vi "Configuration Window.vi"(8 "error in (no error)":errorcluster, 11 "DB Ref":refnum<class "SharedData.lvclass">) -> (0 "error out":errorcluster, 3 "DB Ref (dup)":refnum<class "SharedData.lvclass">)   [LabVIEW 2014]
uses:
  <vilib>/NEVSTOP/Shared Data Library/SharedData/SharedData.lvclass
  <vilib>/NEVSTOP/Shared Data Library/SharedData/SharedData.lvclass/SharedData.ctl
  <vilib>/NEVSTOP/Shared Data Library/SharedData/Data operation/_int32.vi
  <vilib>/NEVSTOP/Shared Data Library/SharedData/Data operation/_variant.vi
  <vilib>/NEVSTOP/Shared Data Library/SharedData/support/_[error50002]Invalid DataType.vi
  <vilib>/NEVSTOP/Shared Data Library/SharedData/support/_[error50001]Can't Found Value.vi
  <vilib>/NEVSTOP/Shared Data Library/SharedData/support/_[error50000]Invalid DB REF.vi
  <vilib>/Utility/error.llb/Trim Whitespace.vi
panel:
  in  "Display Time(ms)":i32 min=0 max=10000 step=100
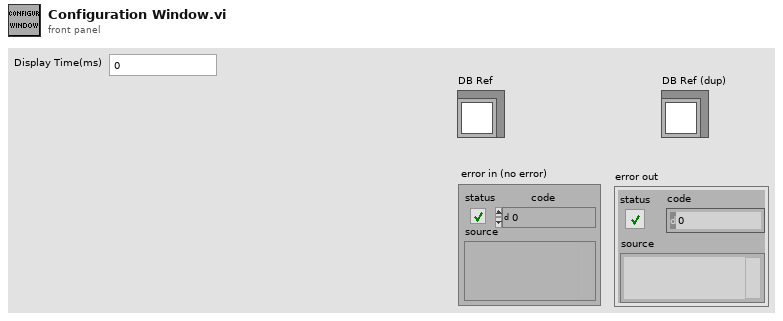
[diagram p1: front panel]
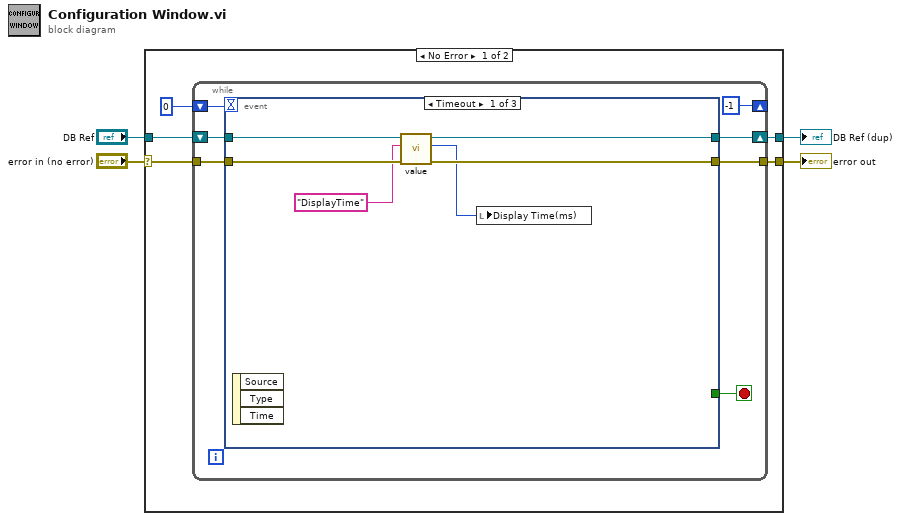
[diagram p0: block diagram]
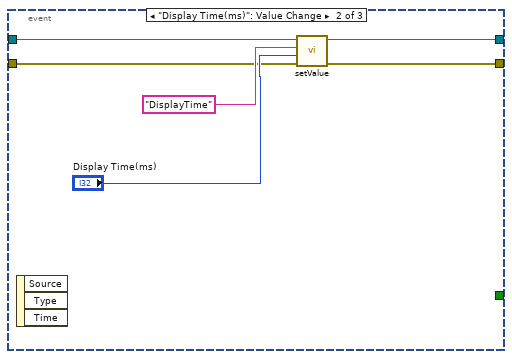
[diagram p2: hidden frame]
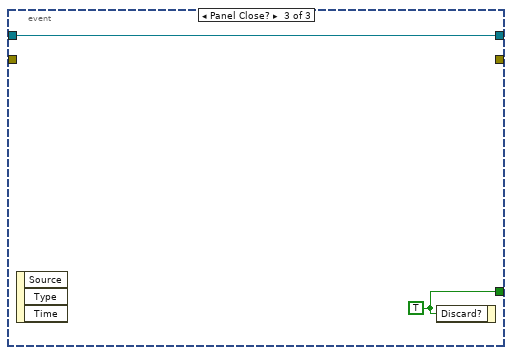
[diagram p3: hidden frame]
diagram:
  n1 = case shown="No Error" "error in (no error)" {
    selector: "error in (no error)" -> [w6 w32]
    tunnel: [w5 w32] -> w3
    tunnel: [w8 w31] -> w2
    tunnel: "DB Ref" -> [w9 w31]
    frame No Error {
      n2 = while {
        shift-right: [-1] -> _
        shift-left: 0 -> [w14]
        shift-right: [w16] -> w8
        shift-left: w9 -> [w15]
        tunnel: w6 -> [w11]
        tunnel: [w10] -> w5
        stop <- w12 stop-if-true
        n3 = event shown="[0] Timeout" {
          selector: _ -> [_ _ _]
          dyn-events: _ -> [_ _ _]
          timeout: w14 -> [_ _ _]
          tunnel: [w20 w27 w29] -> w16
          tunnel: w15 -> [w22 w28 w29]
          tunnel: [_ _ w30] -> w12
          tunnel: w11 -> [w21 w24 _]
          tunnel: [w19 w23 _] -> w10
          event Timeout {
            n4 = event-data() -> ()  [unwired: 1 in, 3 out]
            n5 = call-poly <vilib>:"value.vi"("error in (no error)"=w21, "name"="DisplayTime", "DB Ref"=w22) -> ("error in (no error) (dup)"=w19:errorcluster, "value"=w17:i32, "DB Ref (dup)"=w20:refnum<class "SharedData.lvclass">)  [unwired: 6 in]
            n6 = local write "Display Time(ms)"(w17) -> ()
          }
          event "Display Time(ms)": Value Change {
            n7 = event-data() -> ()  [unwired: 1 in, 3 out]
            n8 = call <vilib>:"setValue.vi"("error in (no error)"=w24, "value"="Display Time(ms)", "name"="DisplayTime", "DB Ref"=w28) -> ("error in (no error) (dup)"=w23:errorcluster, "DB Ref (dup)"=w27:refnum<class "SharedData.lvclass">)  [unwired: 5 in, 1 out]
          }
          event Panel Close? {
            w30 = TRUE
            n9 = event-data() -> ()  [unwired: 1 in, 3 out]
            n10 = event-data("Discard?"=w30) -> ()  [unwired: 1 in, 1 out]
          }
        }
      }
    }
    frame Error {
    }
  }
  "DB Ref (dup)" <- w2
  "error out" <- w3
